vi "RobotDemo.vi"() -> ()   [LabVIEW 2012]
uses:
  <userlib>/rosforlv/Gazebo/URDF_conversion/JointTypes.ctl
panel:
  out "3D Picture":refnum<vi>(3d-picture)
  out "urdf out":string
  # "`"
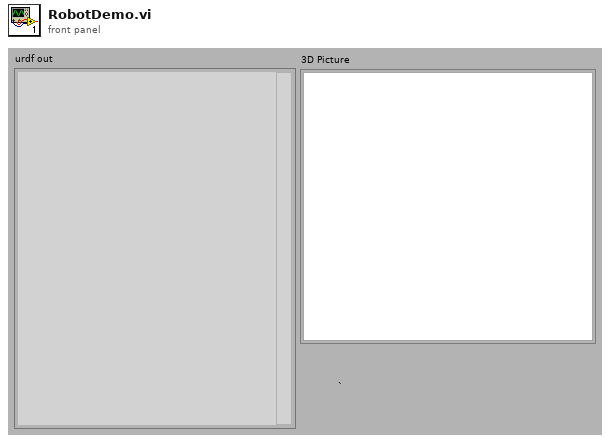
[diagram p1: front panel]
types:
  T1 = typedef "JointTypes.ctl" = enum16{"revolute", "continuous", "prismatic", "fixed", "floating", "planar"}
  T2 = cluster{"Joint Name":string, "type":T1, "axis":enum16{"X", "Y", "Z"}}
  T3 = cluster{"X":sgl, "Y":sgl, "Z":sgl, "roll":sgl, "pitch":sgl, "yaw":sgl}
  T4 = typedef "LINK.ctl" = cluster{"Name":string, "urdf":string}
  T5 = typedef "JOINT.ctl" = cluster{"Joint Name":string, "type":T1, "urdf ":string, "Links":T4[]}
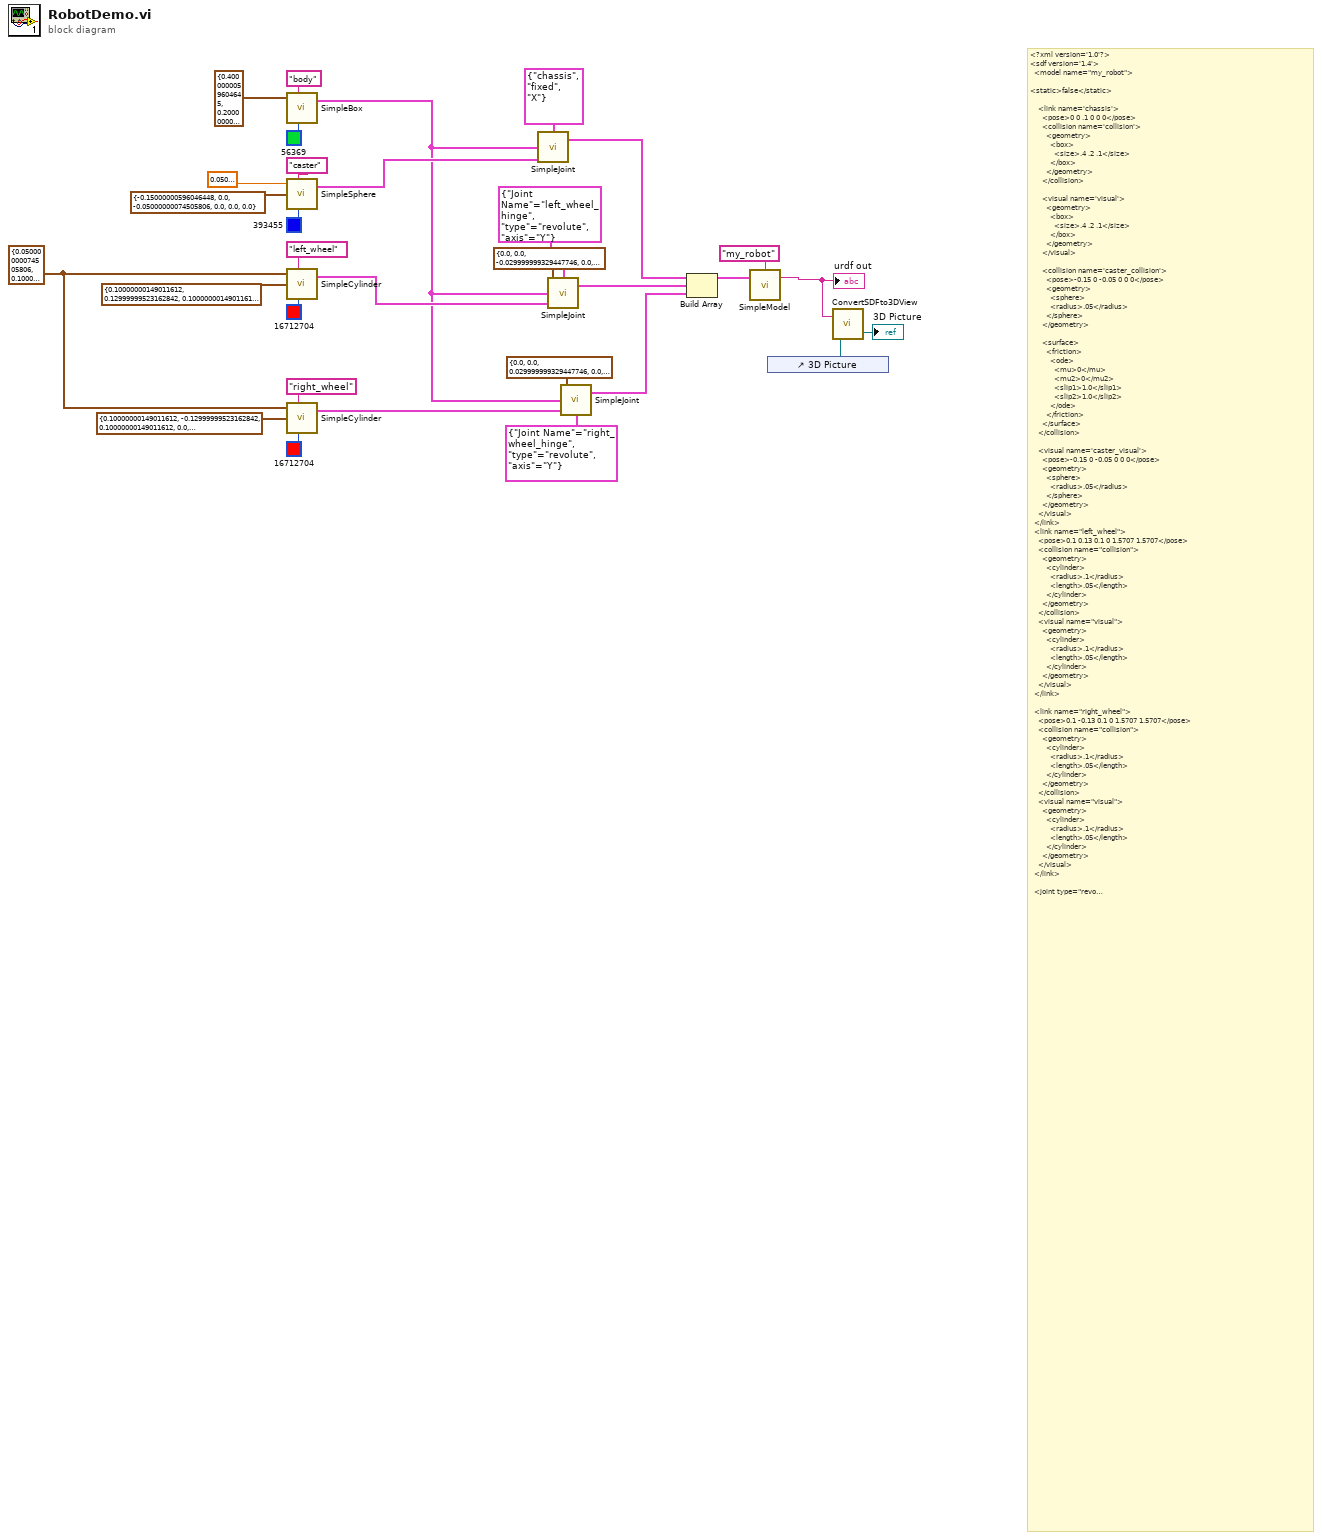
[diagram p0: block diagram]
diagram:
  w15 = cluster{"Length":sgl, "Radius":sgl} {"Length"=0.05, "Radius"=0.1} ("Cylinder")
  # "<?xml version='1.0'?>\n<sdf version='1.4'>\n  <model name=\"my_robot\">\n\n<static>false</static>\n\n    <link name='chassis'>\n      <pose>0 0 .1 0 0 0</pose>\n      <collision name='collision'>\n        <geometry>\n          <box>\n            <size>.4 .2 .1</size>\n          </box>\n        </geometry>\n      </collision>\n\n      <visual name='visual'>\n        <geometry>\n          <box>\n            <size>.4 .2 .1</size>\n          </box>\n        </geometry>\n      </visual>\n\n      <collision name='caster_collision'>\n        <pose>-0.15 0 -0.05 0 0 0</pose>\n        <geometry>\n          <sphere>\n          <radius>.05</radius>\n        </sphere>\n      </geometry>\n\n      <surface>\n        <friction>\n          <ode>\n            <mu>0</mu>\n            <mu2>0</mu2>\n            <slip1>1.0</slip1>\n            <slip2>1.0</slip2>\n          </ode>\n        </friction>\n      </surface>\n    </collision>\n\n    <visual name='caster_visual'>\n      <pose>-0.15 0 -0.05 0 0 0</pose>\n      <geometry>\n        <sphere>\n          <radius>.05</radius>\n        </sphere>\n      </geometry>\n    </visual>\n  </link>     \n  <link name=\"left_wheel\">\n    <pose>0.1 0.13 0.1 0 1.5707 1.5707</pose>\n    <collision name=\"collision\">\n      <geometry>\n        <cylinder>\n          <radius>.1</radius>\n          <length>.05</length>\n        </cylinder>\n      </geometry>\n    </collision>\n    <visual name=\"visual\">\n      <geometry>\n        <cylinder>\n          <radius>.1</radius>\n          <length>.05</length>\n        </cylinder>\n      </geometry>\n    </visual>\n  </link>\n\n  <link name=\"right_wheel\">\n    <pose>0.1 -0.13 0.1 0 1.5707 1.5707</pose>\n    <collision name=\"collision\">\n      <geometry>\n        <cylinder>\n          <radius>.1</radius>\n          <length>.05</length>\n        </cylinder>\n      </geometry>\n    </collision>\n    <visual name=\"visual\">\n      <geometry>\n        <cylinder>\n          <radius>.1</radius>\n          <length>.05</length>\n        </cylinder>\n      </geometry>\n    </visual>\n  </link>\n\n  <joint type=\"revolute\" name=\"left_wheel_hinge\">\n    <pose>0 0 -0.03 0 0 0</pose>\n    <child>left_wheel</child>\n    <parent>chassis</parent>\n    <axis>\n      <xyz>0 1 0</xyz>\n    </axis>\n  </joint>\n\n  <joint type=\"revolute\" name=\"right_wheel_hinge\">\n    <pose>0 0 0.03 0 0 0</pose>\n    <child>right_wheel</child>\n    <parent>chassis</parent>\n    <axis>\n      <xyz>0 1 0</xyz>\n    </axis>\n  </joint>\n\n  </model>\n</sdf>"
  n1 = call <userlib>:"SimpleBox.vi"("Box"=cluster{"Length":sgl, "Width":sgl, "Height":sgl} {"Length"=0.4, "Width"=0.2, "Height"=0.1}, "Name"="body", "link color"=u32 56369) -> ("Link"=w5:T4)  [unwired: 3 in]
  n2 = call <userlib>:"SimpleSphere.vi"("Radius"=sgl 0.05, "Name"="caster", "origin"=T3 {"X"=-0.15, "Y"=0.0, "Z"=-0.05, "roll"=0.0, "pitch"=0.0, "yaw"=0.0} ("Pose"), "link color"=u32 393455) -> ("Link"=w20:T4)  [unwired: 2 in]
  n3 = call <userlib>:"SimpleCylinder.vi"("Cylinder"=w15, "Name"="left_wheel", "origin"=T3 {"X"=0.1, "Y"=0.13, "Z"=0.1, "roll"=0.0, "pitch"=1.57, "yaw"=1.57} ("Pose"), "link color"=u32 16712704) -> ("Link"=w6:T4)  [unwired: 2 in]
  n4 = call <userlib>:"SimpleCylinder.vi"("Cylinder"=w15, "Name"="right_wheel", "origin"=T3 {"X"=0.1, "Y"=-0.13, "Z"=0.1, "roll"=0.0, "pitch"=1.57, "yaw"=1.57} ("Pose"), "link color"=u32 16712704) -> ("Link"=w4:T4)  [unwired: 2 in]
  n5 = call <userlib>:"SimpleJoint.vi"("Joint"=T2 {"Joint Name"="chassis", "type"=enum."fixed", "axis"=enum."X"}, "Child Link"=w20, "Parent Link"=w5) -> ("Joint"=w9:T5)  [unwired: 2 in]
  n6 = call <userlib>:"SimpleJoint.vi"("Joint"=T2 {"Joint Name"="left_wheel_hinge", "type"=enum."revolute", "axis"=enum."Y"}, "Child Link"=w6, "Parent Link"=w5, "origin"=T3 {"X"=0.0, "Y"=0.0, "Z"=-0.03, "roll"=0.0, "pitch"=0.0, "yaw"=0.0} ("Pose")) -> ("Joint"=w8:T5)  [unwired: 1 in]
  n7 = call <userlib>:"SimpleJoint.vi"("Joint"=T2 {"Joint Name"="right_wheel_hinge", "type"=enum."revolute", "axis"=enum."Y"}, "Child Link"=w4, "Parent Link"=w5, "origin"=T3 {"X"=0.0, "Y"=0.0, "Z"=0.03, "roll"=0.0, "pitch"=0.0, "yaw"=0.0} ("Pose")) -> ("Joint"=w7:T5)  [unwired: 1 in]
  n8 = Build Array(w9, w8, w7) -> (w3:T5[])
  n9 = call <userlib>:"SimpleModel.vi"("Joints"=w3, "Name"="my_robot") -> ("urdf out"=w1:string)  [unwired: 2 in]
  "urdf out" <- w1
  n10 = control-ref of="3D Picture"() -> (w28:refnum<vi>)
  n11 = call <userlib>:"ConvertSDFto3DView.vi"("SceneGraphDisp Refnum"=w28, "urdf"=w1) -> ("3D Picture"=→"3D Picture":refnum<vi>)  [unwired: 1 out]
